vi "FTW-Message-Reply.vi"(0 "FTW Incoming Message":refnum<class "FTW-Message.lvclass">, 5 "Response":string, 7 "Send Timeout":i32 format="%dmsec", 11 "error in":errorcluster) -> (6 "Timed out?":bool, 15 "error out":errorcluster)   [LabVIEW 2013, in "FTW-Message.lvclass"]
uses:
  FTW-Message.lvclass
  FTW-Message.lvclass/FTW-Message.ctl
  error/FTW-ERR-ThrowGenericError.vi
  error/FTW-ERR-ThrowError.vi
  error/FTW-ERR-CallChain.vi
  string/FTW-STR-ReplaceWhitespace.vi
  socket/FTW-Socket.lvclass
panel:
  # "Inputs"
  # "Outputs"
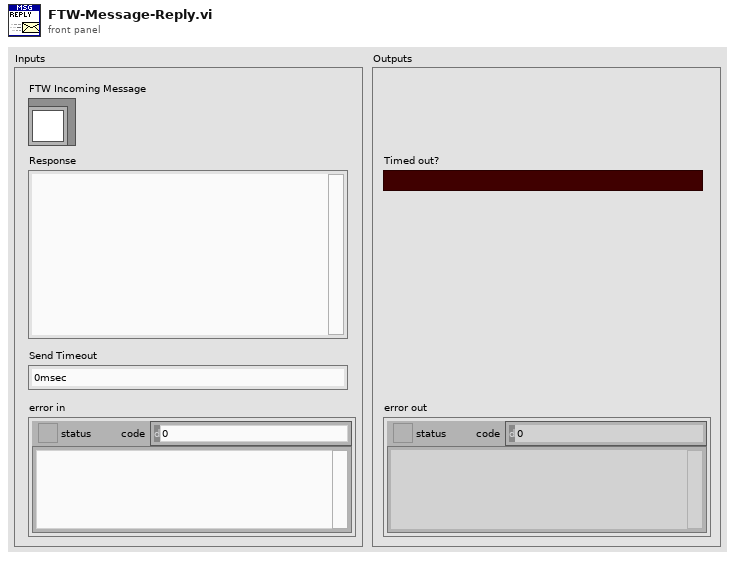
[diagram p1: front panel]
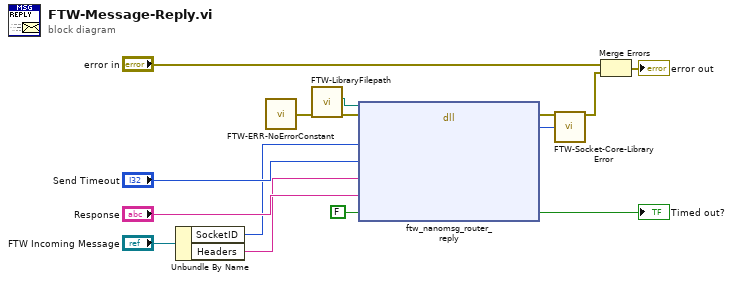
[diagram p0: block diagram]
diagram:
  n1 = Unbundle By Name("FTW Incoming Message") -> ("SocketID"=w5:i64, "Headers"=w4:string)
  n2 = call "FTW-ERR-NoErrorConstant.vi"() -> ("no error"=w9:errorcluster)
  n3 = call "FTW-LibraryFilepath.vi"("error in"=w9) -> ("error out"=w13:errorcluster, "Library Filepath"=w1:path)  [unwired: 8 in, 1 out]
  n4 = dll-call lib="?" fn="ftw_nanomsg_router_reply"(path in=w1, error in=w13, "RouterID"=w5, "Timeout"="Send Timeout", "Backtrace"=w4, "Response"="Response", "Timed out?"=FALSE) -> (error out=w11:errorcluster, "Return Value"=w12:i64, "Timed out?"=→"Timed out?":bool)  [unwired: 5 in, 1 out]
  n5 = call "FTW-Socket-Core-LibraryError.vi"("error in"=w11, "Return Value"=w12) -> ("error out"=w8:errorcluster)  [unwired: 13 in]
  n6 = Merge Errors("error in", w8) -> (→"error out":errorcluster)
